vi "Multi Data Processor.vi"(8 "error in (no error)":errorcluster, 11 "Synapse CCD.lvclass In":refnum<class "Synapse CCD.lvclass">) -> (0 "error out":errorcluster, 1 "Processed Array":dbl[](array[numeric]), 2 "Processed Spectrum":cluster{"Ramp Pattern":dbl[], "X array":dbl[]}[](graph), 3 "Synapse CCD.lvclass Out":refnum<class "Synapse CCD.lvclass">)   [LabVIEW 2015, in "Synapse CCD.lvclass"]
doc: "Processes Multi-Data based on member data Booleans. Returns Single Spectrum Plot and stores data in member data.\n\nPossible options include:\n\nDark Subtraction\nAveraging Multiple Scans\nCosmic Ray Removal"
uses:
  Synapse CCD.lvclass
  Synapse CCD.lvclass/Synapse CCD.ctl
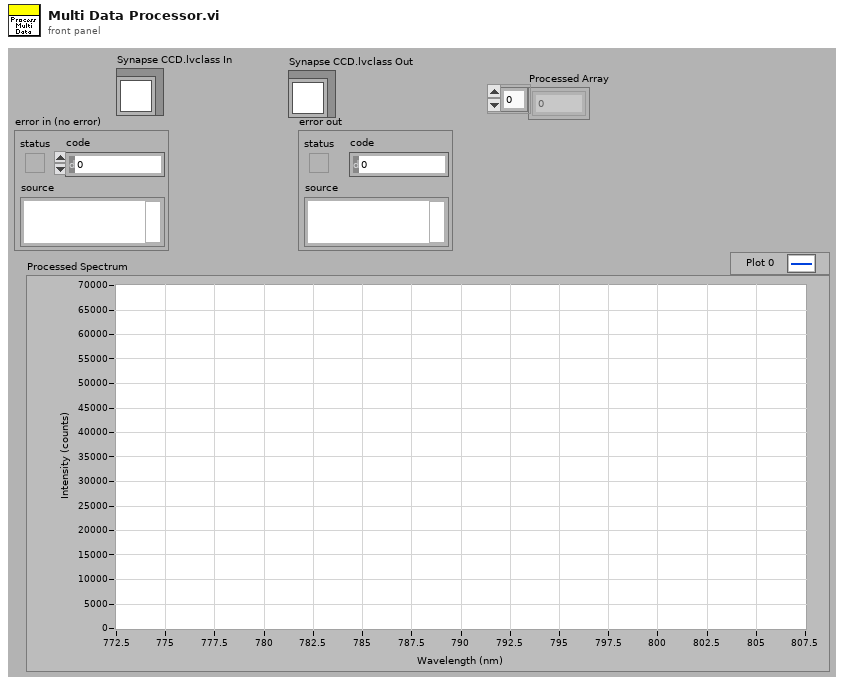
[diagram p1: front panel]
types:
  T1 = cluster{"Array of Wavelengths":dbl[], "Processed Data":dbl[]}
  T2 = cluster{"Array of Wavelengths":dbl[], "Processed Data":dbl[]}[]
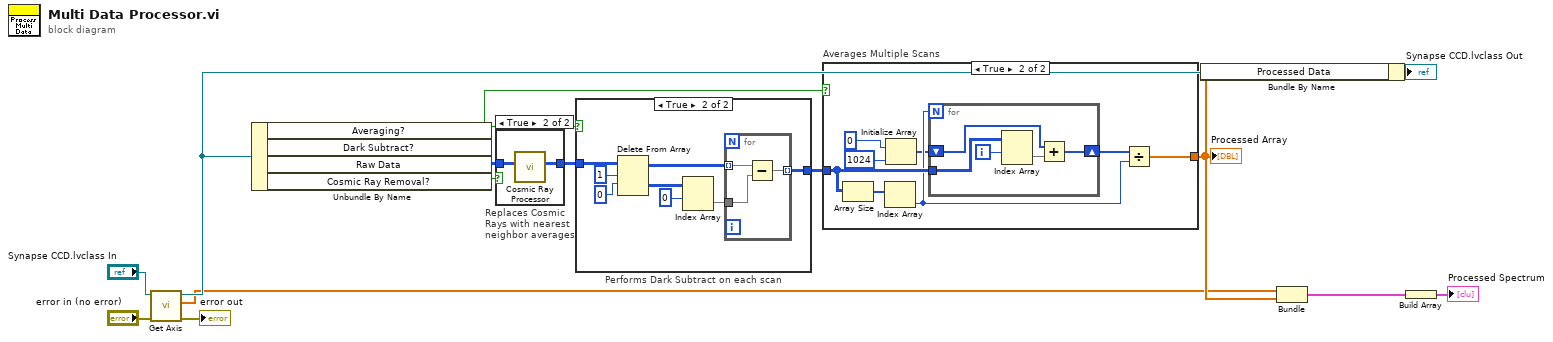
[diagram p0: block diagram]
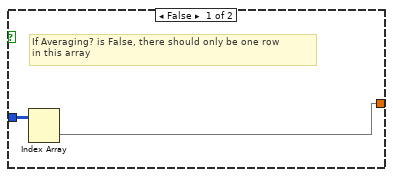
[diagram p3: hidden frame]
diagram:
  n1 = call "Get Axis.vi"("error in (no error)"="error in (no error)", "Synapse CCD.lvclass In"="Synapse CCD.lvclass In") -> ("error out"=→"error out":errorcluster, "Array of Wavelengths"=w4:dbl[], "Synapse CCD.lvclass Out"=w8:refnum<class "Synapse CCD.lvclass">)  [unwired: 7 in]
  n2 = Unbundle By Name(w8) -> ("Averaging?"=w13:bool, "Dark Subtract?"=w14:bool, "Raw Data"=w2:i32[][], "Cosmic Ray Removal?"=w3:bool)
  n3 = case "Replaces Cosmic\nRays with nearest\nneighbor averages" shown="True" w3 {
    tunnel: w2 -> [w16 w18]
    tunnel: [w16 w17] -> w1
    frame False {
    }
    frame True {
      n4 = call "Cosmic Ray Processor.vi"("Raw Data"=w18) -> ("Processed Data"=w17:i32[][])  [unwired: 10 in]
    }
  }
  n5 = case "Performs Dark Subtract on each scan" shown="True" w14 {
    tunnel: w1 -> [w19 w24]
    tunnel: [w19 w21] -> w15
    frame False {
    }
    frame True {
      n6 = Delete From Array(array=w24, length=1, index (row)=0) -> (deleted portion=w20:i32[][], array with subset deleted=w25:i32[][])  [unwired: 1 in]
      n7 = Index Array(array=w20, index (row)=0) -> (element=w22:i32[])  [unwired: 1 in]
      n8 = for {
        tunnel: w25 -> [w30] mode=indexing
        tunnel: w22 -> [w29]
        tunnel: [w28] -> w21 mode=indexing
        n9 = Subtract(x=w30, y=w29) -> (x-y=w28:i32[])
      }
    }
  }
  n10 = case "Averages Multiple Scans" shown="True" w13 {
    tunnel: w15 -> [w32 w39]
    tunnel: [w31 w36] -> w5
    frame False {
      # "If Averaging? is False, there should only be one row\nin this array"
      n11 = Index Array(array=w32) -> (element=w31:i32[])  [unwired: 2 in]
    }
    frame True {
      n12 = Array Size(array=w39) -> (size(s)=w40:i32[])
      n13 = Index Array(array=w40) -> (element=w37:i32)  [unwired: 1 in]
      n14 = Initialize Array(0, 1024) -> (w33:i32[])
      n15 = for {
        N: w37 -> [_]
        tunnel: w39 -> [w43]
        shift-right: [w41] -> w38
        shift-left: w33 -> [w45]
        i -> [w44]
        n16 = Index Array(array=w43, index (row)=w44) -> (element=w42:i32[])  [unwired: 1 in]
        n17 = Add(x=w45, y=w42) -> (x+y=w41:i32[])
      }
      n18 = Divide(x=w38, y=w37) -> (x/y=w36:dbl[])
    }
  }
  "Processed Array" <- w5
  n19 = Bundle By Name(cluster=w8, "Processed Data"=w5) -> (→"Synapse CCD.lvclass Out":refnum<class "Synapse CCD.lvclass">)
  n20 = Bundle("Array of Wavelengths"=w4, "Processed Data"=w5) -> (w7:T1)  [unwired: 1 in]
  n21 = Build Array(w7) -> (→"Processed Spectrum":T2)
